vi "MEMS_InitDevice.vi"(7 "ComCluster in":T11, 8 "C_Motion":T1={"Task"=enum."Init", "C_Waveform_Par"={"A-Scan_Rate"=0.0, "A-Scans"=0, "B-Scans"=0, "B-Scan_Avg."=0, "x_min"=0.0, "x_max"=0.0, "y_min"=0.0, "y_max"=0.0, "B_Switch_Dir"=FALSE, "Divider"=0.0, "Up_only"=FALSE, "Phase shift [Pixel]"=0.0, "Scale Factor [mm/V]"=1.0, "E_Scanner"=enum."MEMS"}} {"C_Waveform_Par"."A-Scan_Rate" min=1.0 max=100000.0}, 9 "SignalInfo out":T7={"AScanPerBScan"=0.0, "BScanPerCScan"=0.0, "FastAxis"=enum."X-Axis", "SlowAxis"=enum."X-Axis", "FastAxisFilter"=enum."NoFilter", "SlowAxisFilter"=enum."NoFilter", "AmpFastAxis"=0.0, "AmpSlowAxis"=0.0}, 10 "MCU_Config out":T10) -> (0 "error out":errorcluster, 1 "SignalInfo out 2":T7={"AScanPerBScan"=0.0, "BScanPerCScan"=0.0, "FastAxis"=enum."X-Axis", "SlowAxis"=enum."X-Axis", "FastAxisFilter"=enum."NoFilter", "SlowAxisFilter"=enum."NoFilter", "AmpFastAxis"=0.0, "AmpSlowAxis"=0.0}, 2 "MCU_Config out 2":T10, 5 "ComCluster in 2":T11)   [LabVIEW 2019]
uses:
  OCTTypeTypeDef.ctl
  ScanningModeTypeDef.ctl
  OutputStageTypeDef.ctl
  FilterTypeDef.ctl
  common-oct-library/TypeDefs/C_Motion.ctl
  common-oct-library/TypeDefs/E_Motion.ctl
  common-oct-library/TypeDefs/C_Waveform_Par.ctl
  common-oct-library/TypeDefs/E_Scanner.ctl
  MEMS_CmdsTypeDef.ctl
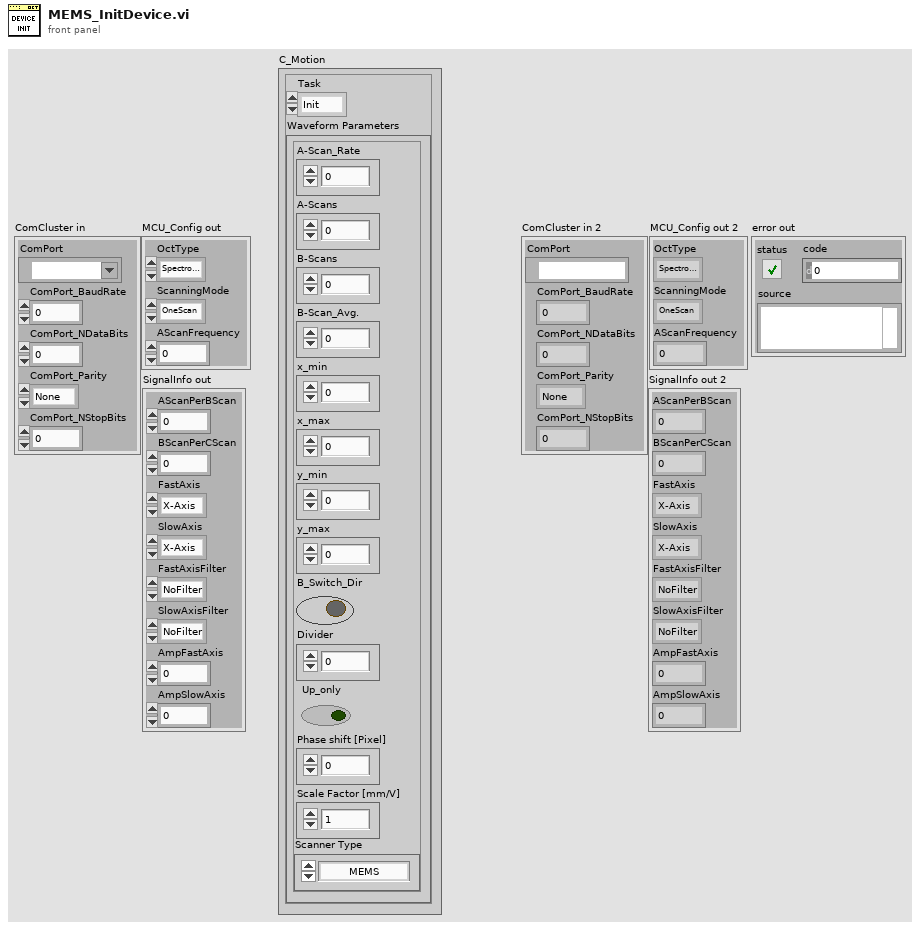
[diagram p1: front panel]
types:
  T1 = typedef "C_Motion.ctl" = cluster{"Task":T2, "C_Waveform_Par":T3}
  T2 = typedef "E_Motion.ctl" = enum16{"Init", "Init-Device", "Start-Device", "Stop-Device", "Error", "Done"}
  T3 = typedef "C_Waveform_Par.ctl" = cluster{"A-Scan_Rate":dbl, "A-Scans":i32, "B-Scans":i32, "B-Scan_Avg.":i32, "x_min":dbl, "x_max":dbl, "y_min":dbl, "y_max":dbl, "B_Switch_Dir":bool, "Divider":dbl, "Up_only":bool, "Phase shift [Pixel]":dbl, "Scale Factor [mm/V]":dbl, "E_Scanner":T4}
  T4 = typedef "E_Scanner.ctl" = enum16{"Galvo ", "MEMS", "No Sanner"}
  T5 = typedef "OutputStageTypeDef.ctl" = enum16{"X-Axis", "Y-Axis"}
  T6 = typedef "FilterTypeDef.ctl" = enum16{"IIR_Slow", "IIR_Fast", "NoFilter", "Bessel6thOrder300"}
  T7 = cluster{"AScanPerBScan":dbl, "BScanPerCScan":dbl, "FastAxis":T5, "SlowAxis":T5, "FastAxisFilter":T6, "SlowAxisFilter":T6, "AmpFastAxis":dbl, "AmpSlowAxis":dbl}
  T8 = typedef "OCTTypeTypeDef.ctl" = enum16{"Spectrometer OCT", "SSOCT"}
  T9 = typedef "ScanningModeTypeDef.ctl" = enum16{"OneScan", "ContinuousScan"}
  T10 = cluster{"OctType":T8, "ScanningMode":T9, "AScanFrequency":dbl}
  T11 = cluster{"ComPort":refnum<visa-resource-name>, "ComPort_BaudRate":u32, "ComPort_NDataBits":u16, "ComPort_Parity":enum16{"None", "Odd", "Even", "Mark", "Space"}, "ComPort_NStopBits":u16}
  T12 = typedef "MEMS_CmdsTypeDef.ctl" = enum16{"Init", "Config_AScan", "Config_BScan", "Config_CScan", "Run", "Stop", "Shutdown"}
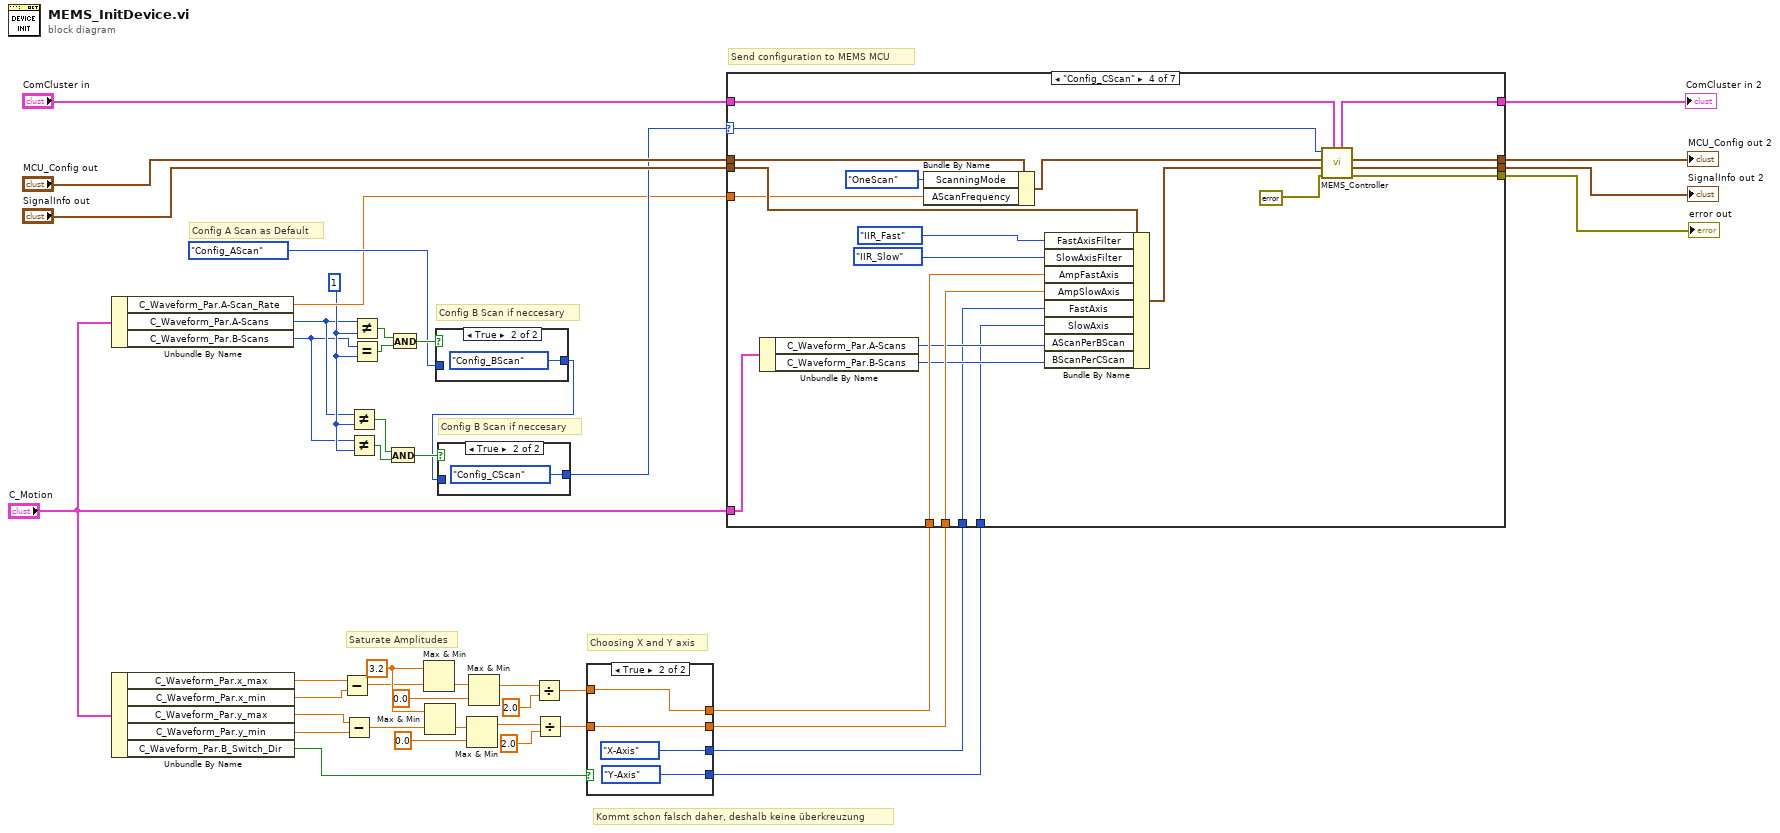
[diagram p0: block diagram]
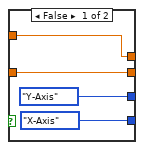
[diagram p4: hidden frame]
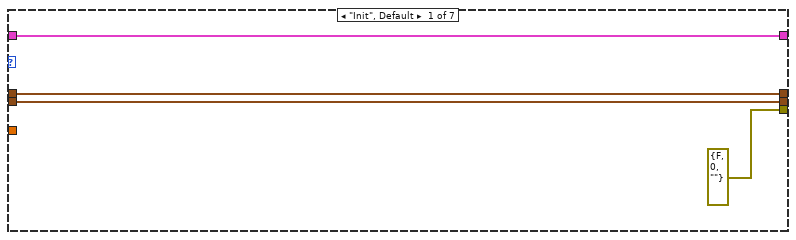
[diagram p5: hidden frame]
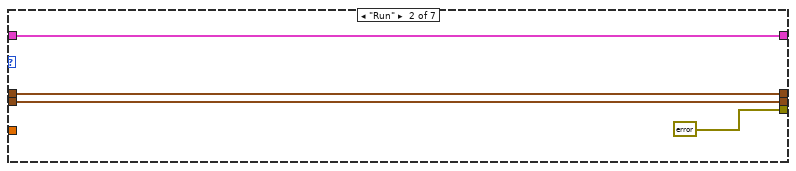
[diagram p6: hidden frame]
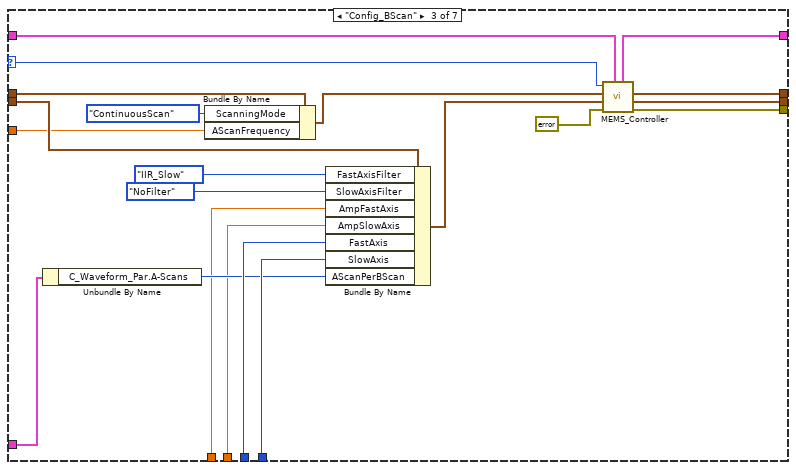
[diagram p7: hidden frame]
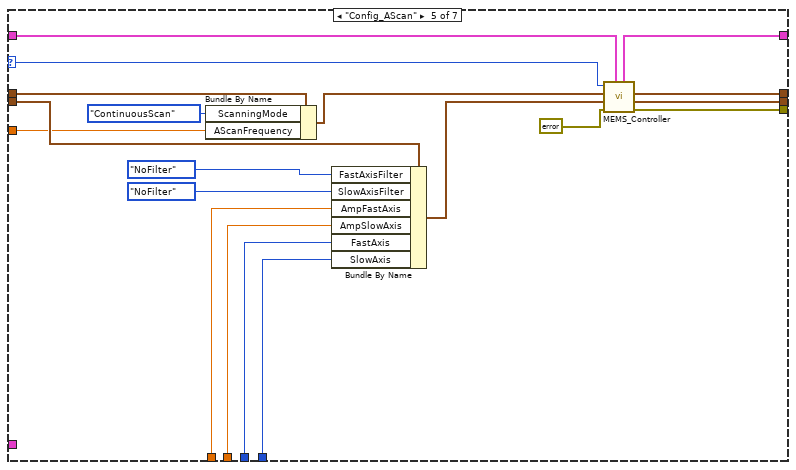
[diagram p8: hidden frame]
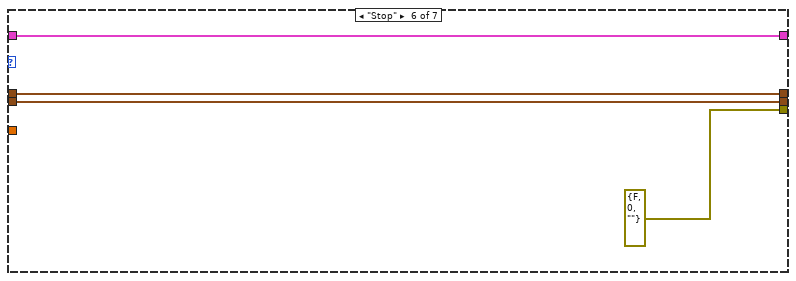
[diagram p9: hidden frame]
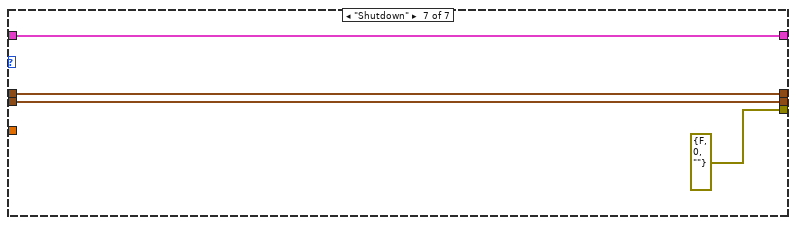
[diagram p10: hidden frame]
diagram:
  w8 = 1 ("x")
  w36 = 3.2 ("x")
  # "Kommt schon falsch daher, deshalb keine überkreuzung"
  # "Send configuration to MEMS MCU"
  # "Config B Scan if neccesary"
  # "Config A Scan as Default"
  # "Config B Scan if neccesary"
  # "Choosing X and Y axis"
  # "Saturate Amplitudes"
  n1 = Unbundle By Name("C_Motion") -> ("C_Waveform_Par.A-Scan_Rate"=w17:dbl, "C_Waveform_Par.A-Scans"=w7:i32, "C_Waveform_Par.B-Scans"=w6:i32)
  n2 = Unbundle By Name("C_Motion") -> ("C_Waveform_Par.x_max"=w27:dbl, "C_Waveform_Par.x_min"=w26:dbl, "C_Waveform_Par.y_max"=w25:dbl, "C_Waveform_Par.y_min"=w24:dbl, "C_Waveform_Par.B_Switch_Dir"=w23:bool)
  n3 = Subtract(x=w27, y=w26) -> (x-y=w31:dbl)
  n4 = Subtract(x=w25, y=w24) -> (x-y=w30:dbl)
  n5 = Not Equal?(x=w7, y=w8) -> (x != y?=w5:bool)
  n6 = Not Equal?(x=w6, y=w8) -> (x != y?=w4:bool)
  n7 = Not Equal?(x=w7, y=w8) -> (x != y?=w10:bool)
  n8 = Equal?(x=w6, y=w8) -> (x = y?=w9:bool)
  n9 = And(x=w5, y=w4) -> (x .and. y?=w20:bool)
  n10 = And(x=w10, y=w9) -> (x .and. y?=w22:bool)
  n11 = Max & Min(x=w36, y=w31) -> (min(x,y)=w39:dbl)  [unwired: 1 out]
  n12 = Max & Min(x=w36, y=w30) -> (min(x,y)=w37:dbl)  [unwired: 1 out]
  n13 = case shown="True" w22 {
    tunnel: MEMS_CmdsTypeDef."Config_AScan" ("MEMS_Cmds") -> [w44 _]
    tunnel: [w44 MEMS_CmdsTypeDef."Config_BScan" ("MEMS_Cmds")] -> w19
    frame False {
    }
    frame True {
    }
  }
  n14 = case shown="True" w20 {
    tunnel: w19 -> [w46 _]
    tunnel: [w46 MEMS_CmdsTypeDef."Config_CScan" ("MEMS_Cmds")] -> w18
    frame False {
    }
    frame True {
    }
  }
  n15 = Max & Min(x=w37, y=0.0) -> (max(x,y)=w33:dbl)  [unwired: 1 out]
  n16 = Max & Min(x=w39, y=0.0) -> (max(x,y)=w35:dbl)  [unwired: 1 out]
  n17 = Divide(x=w35, y=2.0) -> (x/y=w29:dbl)
  n18 = Divide(x=w33, y=2.0) -> (x/y=w28:dbl)
  n19 = case shown="True" w23 {
    tunnel: [OutputStageTypeDef."Y-Axis" ("FastAxis") OutputStageTypeDef."X-Axis" ("FastAxis")] -> w2
    tunnel: [OutputStageTypeDef."X-Axis" ("FastAxis") OutputStageTypeDef."Y-Axis" ("FastAxis")] -> w1
    tunnel: w28 -> [w48 w52]
    tunnel: w29 -> [w49 w53]
    tunnel: [w49 w53] -> w16
    tunnel: [w48 w52] -> w15
    frame False {
    }
    frame True {
    }
  }
  n20 = case shown="\"Config_CScan\"" w18 {
    selector: w18 -> [_ _ w68 w90 w109 _ _]
    tunnel: "ComCluster in" -> [w59 w63 w66 w89 w108 w129 w133]
    tunnel: "MCU_Config out" -> [w58 w62 w78 w101 w119 w128 w132]
    tunnel: "SignalInfo out" -> [w57 w61 w77 w100 w118 w127 w131]
    tunnel: [w59 w63 w67 w88 w107 w129 w133] -> w14
    tunnel: [w58 w62 w73 w96 w116 w128 w132] -> w13
    tunnel: [w57 w61 w72 w95 w115 w127 w131] -> w12
    tunnel: w17 -> [_ _ w76 w99 w117 _ _]
    tunnel: [errorcluster {"status"=FALSE, "code"=0, "source"=""} ("error out") errorcluster {"status"=FALSE, "code"=0, "source"=""} ("error out") w71 w94 w114 errorcluster {"status"=FALSE, "code"=0, "source"=""} ("error out") errorcluster {"status"=FALSE, "code"=0, "source"=""} ("error out")] -> w11
    tunnel: w2 -> [_ _ w75 w86 w112 _ _]
    tunnel: w1 -> [_ _ w74 w87 w113 _ _]
    tunnel: w16 -> [_ _ w65 w98 w111 _ _]
    tunnel: w15 -> [_ _ w64 w97 w110 _ _]
    tunnel: "C_Motion" -> [_ _ w70 w93 _ _ _]
    frame "Init", Default {
    }
    frame "Run" {
    }
    frame "Config_BScan" {
      n21 = Unbundle By Name(w70) -> ("C_Waveform_Par.A-Scans"=w69:i32)
      n22 = Bundle By Name(cluster=w78, "ScanningMode"=ScanningModeTypeDef."ContinuousScan", "AScanFrequency"=w76) -> (w81:T10)
      n23 = Bundle By Name(cluster=w77, "FastAxisFilter"=FilterTypeDef."IIR_Slow", "SlowAxisFilter"=FilterTypeDef."NoFilter" ("FastAxisFilter"), "AmpFastAxis"=w65, "AmpSlowAxis"=w64, "FastAxis"=w75, "SlowAxis"=w74, "AScanPerBScan"=w69) -> (w79:T7)
      n24 = call "MEMS_Controller.vi"("ComCluster in"=w66, "error in (no error)"=errorcluster {"status"=FALSE, "code"=0, "source"=""}, "SignalInfo in"=w79, "MCU_Config in"=w81, "MEMS_Cmds"=w68) -> ("error out"=w71:errorcluster, "SignalInfo out"=w72:T7, "MCU_Config out"=w73:T10, "ComCluster out"=w67:T11)  [unwired: 3 in]
    }
    frame "Config_CScan" {
      n25 = Unbundle By Name(w93) -> ("C_Waveform_Par.A-Scans"=w92:i32, "C_Waveform_Par.B-Scans"=w91:i32)
      n26 = Bundle By Name(cluster=w101, "ScanningMode"=ScanningModeTypeDef."OneScan", "AScanFrequency"=w99) -> (w104:T10)
      n27 = Bundle By Name(cluster=w100, "FastAxisFilter"=FilterTypeDef."IIR_Fast", "SlowAxisFilter"=FilterTypeDef."IIR_Slow" ("FastAxisFilter"), "AmpFastAxis"=w98, "AmpSlowAxis"=w97, "FastAxis"=w86, "SlowAxis"=w87, "AScanPerBScan"=w92, "BScanPerCScan"=w91) -> (w102:T7)
      n28 = call "MEMS_Controller.vi"("ComCluster in"=w89, "error in (no error)"=errorcluster {"status"=FALSE, "code"=0, "source"=""}, "SignalInfo in"=w102, "MCU_Config in"=w104, "MEMS_Cmds"=w90) -> ("error out"=w94:errorcluster, "SignalInfo out"=w95:T7, "MCU_Config out"=w96:T10, "ComCluster out"=w88:T11)  [unwired: 3 in]
    }
    frame "Config_AScan" {
      n29 = Bundle By Name(cluster=w119, "ScanningMode"=ScanningModeTypeDef."ContinuousScan", "AScanFrequency"=w117) -> (w122:T10)
      n30 = Bundle By Name(cluster=w118, "FastAxisFilter"=FilterTypeDef."NoFilter", "SlowAxisFilter"=FilterTypeDef."NoFilter" ("FastAxisFilter"), "AmpFastAxis"=w111, "AmpSlowAxis"=w110, "FastAxis"=w112, "SlowAxis"=w113) -> (w120:T7)
      n31 = call "MEMS_Controller.vi"("ComCluster in"=w108, "error in (no error)"=errorcluster {"status"=FALSE, "code"=0, "source"=""}, "SignalInfo in"=w120, "MCU_Config in"=w122, "MEMS_Cmds"=w109) -> ("error out"=w114:errorcluster, "SignalInfo out"=w115:T7, "MCU_Config out"=w116:T10, "ComCluster out"=w107:T11)  [unwired: 3 in]
    }
    frame "Stop" {
    }
    frame "Shutdown" {
    }
  }
  "ComCluster in 2" <- w14
  "MCU_Config out 2" <- w13
  "SignalInfo out 2" <- w12
  "error out" <- w11
